vi "Split_Queue(Subvi).vi"(11 "입력 문자열":string) -> (1 "Split_Queue2_Result":string[](array[string]), 2 "Split_Queue2":string, 3 "Split_Queue3":string, 4 "Split_Queue3_Result":string[](array[string]), 5 "Split_Queue4":string, 6 "Split_Queue4_Result":string[](array[string]))   [LabVIEW 2023]
doc: "'''\n해당 함수는 입력 문자열을 분리하여 Queue2,Queue3,Queue4 값으로 분리하여 해당 Loop에 값을 전달한다. \n'''\nInput: '문자열'\n\nReturn:\n __Queue2: BDDATA(DSPEN, TRXPSEN, TRXCEN, MINTIN, BDTEMP, ENVTEMP, PRESSURE, Number\n __Queue3: SIGDATA\n __Queue4: GPSDATA(1PPS,Latitude,Longitude,Numbero"
panel:
  out "일치 + 문자열의 나머지":string
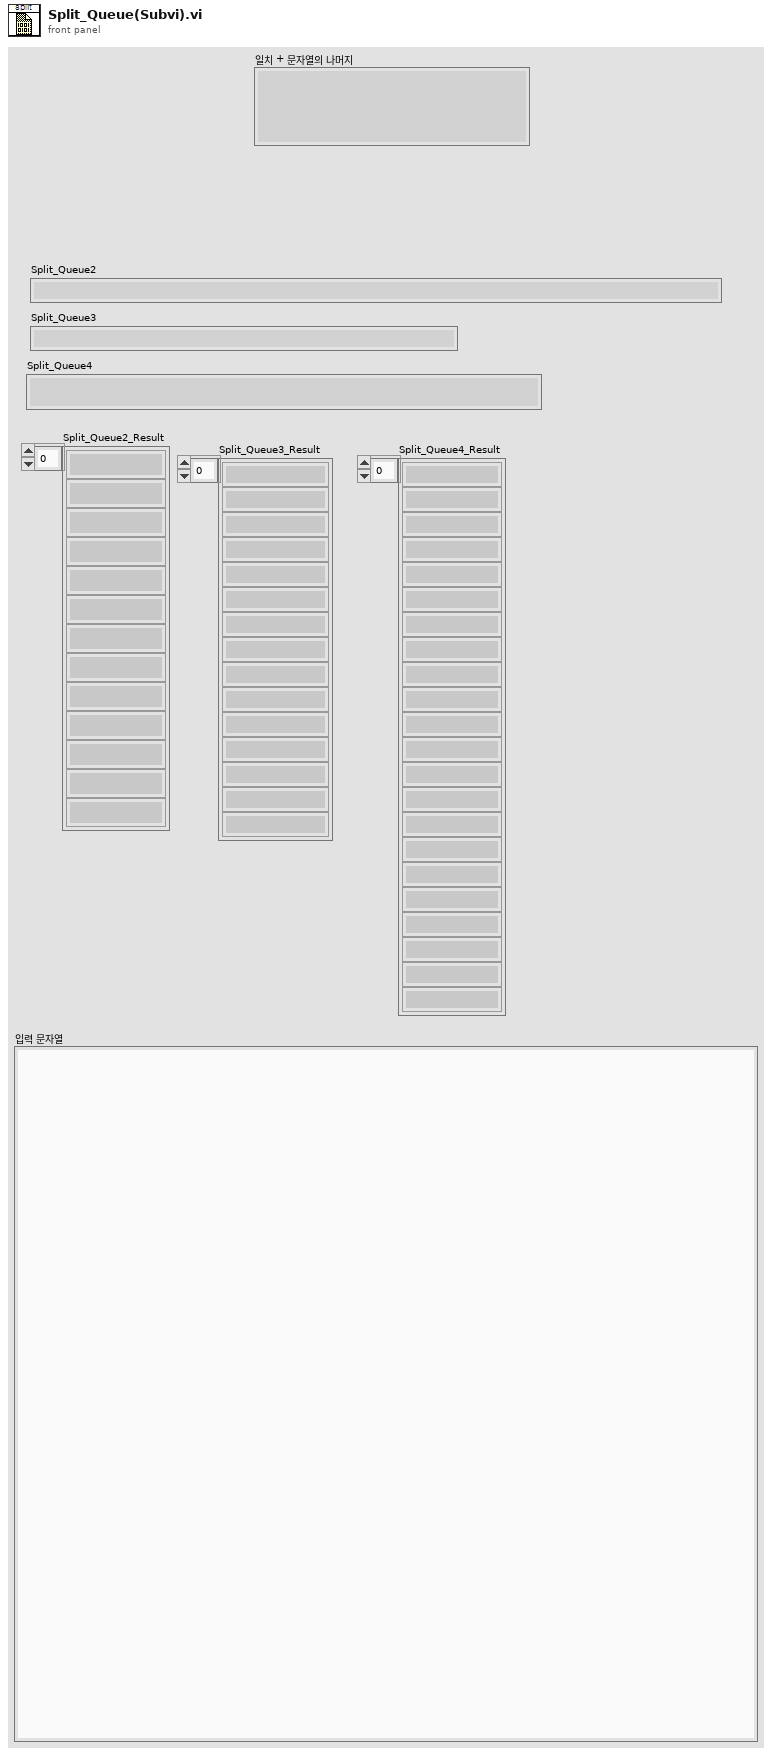
[diagram p1: front panel]
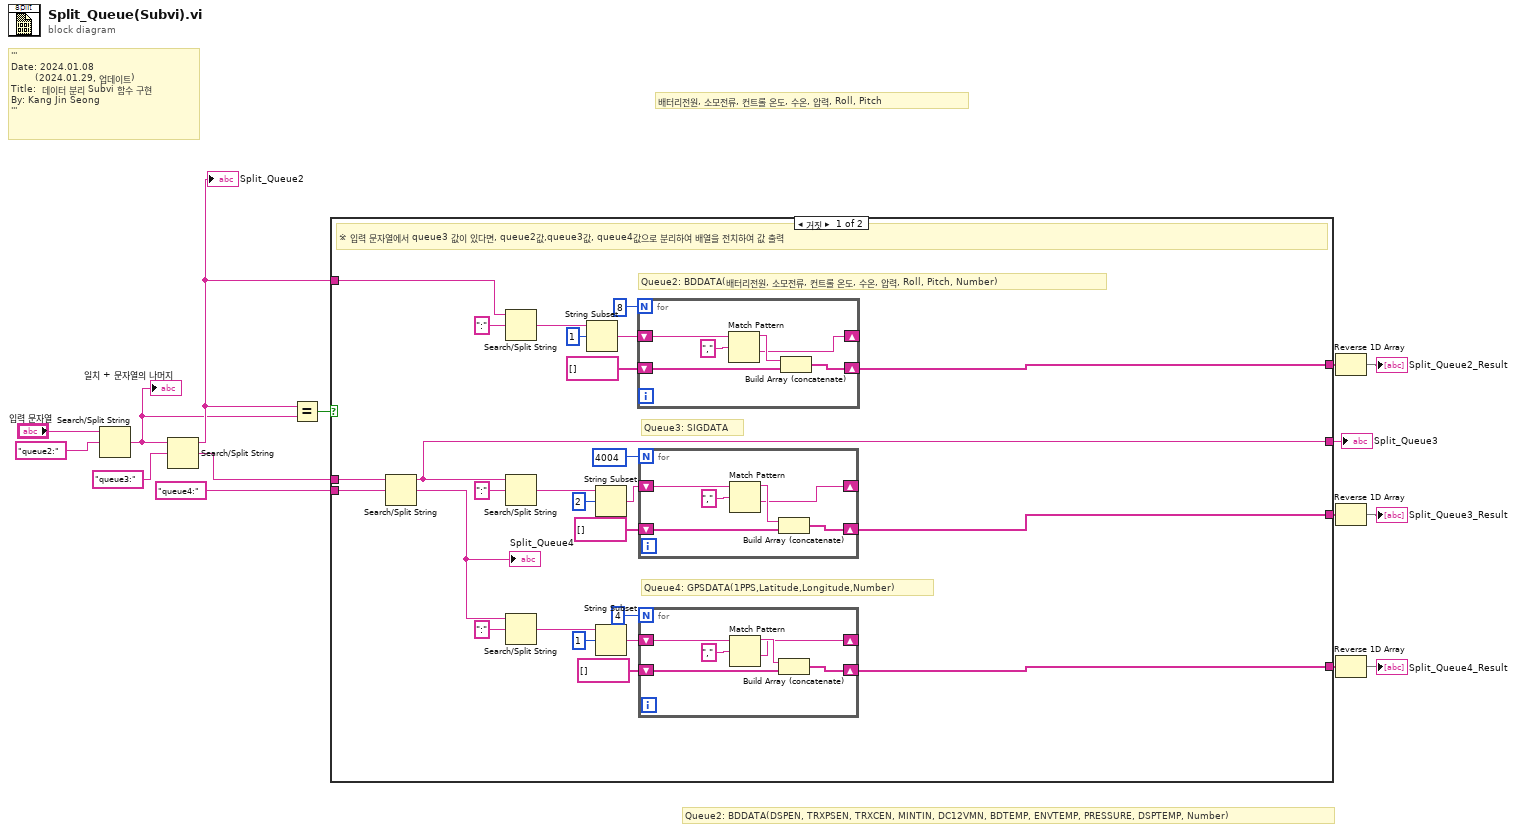
[diagram p0: block diagram]
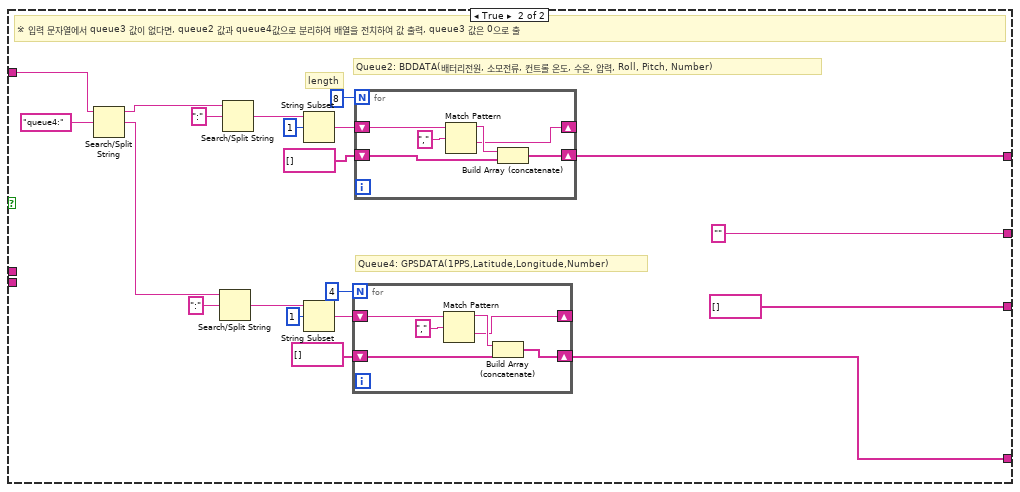
[diagram p2: hidden frame]
diagram:
  # "Queue2: BDDATA(DSPEN, TRXPSEN, TRXCEN, MINTIN, DC12VMN, BDTEMP, ENVTEMP, PRESSURE, DSPTEMP, Number)"
  # "배터리전원, 소모전류, 컨트롤 온도, 수온, 압력, Roll, Pitch"
  # "'''\nDate: 2024.01.08\n        (2024.01.29, 업데이트)\nTitle:  데이터 분리 Subvi 함수 구현\nBy: Kang Jin Seong\n'''"
  n1 = Search/Split String(string="입력 문자열", search string/char (-)="queue2:" ("검색 문자열/문자 (-)")) -> (match + rest of string=w2:string)  [unwired: 1 in, 2 out]
  "일치 + 문자열의 나머지" <- w2
  n2 = Search/Split String(string=w2, search string/char (-)="queue3:" ("검색 문자열/문자 (-)")) -> (substring before match=w3:string, match + rest of string=w7:string)  [unwired: 1 in, 1 out]
  "Split_Queue2" <- w3
  n3 = Equal?(x=w3, y=w2) -> (x = y?=w4:bool)
  n4 = case shown="거짓" w4 {
    tunnel: [w40 w60] -> w13
    tunnel: [w29 string[] []] -> w12
    tunnel: [w28 w69] -> w9
    tunnel: w3 -> [w23 w70]
    tunnel: "queue4:" ("검색 문자열/문자 (-)") -> [w21 _]
    tunnel: w7 -> [w20 _]
    tunnel: [w16 ""] -> w1
    frame False {
      # "Queue2: BDDATA(배터리전원, 소모전류, 컨트롤 온도, 수온, 압력, Roll, Pitch, Number)"
      # "Queue4: GPSDATA(1PPS,Latitude,Longitude,Number)"
      # "Queue3: SIGDATA"
      # "※ 입력 문자열에서 queue3 값이 있다면, queue2값,queue3값, queue4값으로 분리하여 배열을 전치하여 값 출력"
      n5 = Search/Split String(string=w20, search string/char (-)=w21) -> (substring before match=w16:string, match + rest of string=w41:string)  [unwired: 1 in, 1 out]
      "Split_Queue4" <- w41
      n6 = Search/Split String(string=w23, search string/char (-)=":") -> (match + rest of string=w25:string)  [unwired: 1 in, 2 out]
      n7 = Search/Split String(string=w16, search string/char (-)=":") -> (match + rest of string=w32:string)  [unwired: 1 in, 2 out]
      n8 = Search/Split String(string=w41, search string/char (-)=":") -> (match + rest of string=w37:string)  [unwired: 1 in, 2 out]
      n9 = String Subset(string=w25, offset (0)=1 ("오프셋(0)")) -> (substring=w27:string)  [unwired: 1 in]
      n10 = String Subset(string=w32, offset (0)=2 ("오프셋(0)")) -> (substring=w30:string)  [unwired: 1 in]
      n11 = String Subset(string=w37, offset (0)=1 ("오프셋(0)")) -> (substring=w39:string)  [unwired: 1 in]
      n12 = for {
        N: 8 -> [_]
        shift-right: [w56] -> _
        shift-left: w27 -> [w59]
        shift-right: [w55] -> w28
        shift-left: string[] [] -> [w54]
        n13 = Match Pattern(string=w59, regular expression="," ("정규식")) -> (before substring=w57:string, after substring=w56:string)  [unwired: 1 in, 2 out]
        n14 = Build Array (concatenate)(w57, w54) -> (w55:string[])
      }
      n15 = for {
        N: 4004 -> [_]
        shift-right: [w50] -> _
        shift-left: w30 -> [w53]
        shift-right: [w49] -> w29
        shift-left: string[] [] -> [w48]
        n16 = Match Pattern(string=w53, regular expression="," ("정규식")) -> (before substring=w51:string, after substring=w50:string)  [unwired: 1 in, 2 out]
        n17 = Build Array (concatenate)(w51, w48) -> (w49:string[])
      }
      n18 = for {
        N: 4 -> [_]
        shift-right: [w44] -> _
        shift-left: w39 -> [w47]
        shift-right: [w43] -> w40
        shift-left: string[] [] -> [w42]
        n19 = Match Pattern(string=w47, regular expression="," ("정규식")) -> (before substring=w45:string, after substring=w44:string)  [unwired: 1 in, 2 out]
        n20 = Build Array (concatenate)(w45, w42) -> (w43:string[])
      }
    }
    frame True {
      # "length"
      # "Queue2: BDDATA(배터리전원, 소모전류, 컨트롤 온도, 수온, 압력, Roll, Pitch, Number)"
      # "Queue4: GPSDATA(1PPS,Latitude,Longitude,Number)"
      # "※ 입력 문자열에서 queue3 값이 없다면, queue2 값과 queue4값으로 분리하여 배열을 전치하여 값 출력, queue3 값은 0으로 출"
      n21 = Search/Split String(string=w70, search string/char (-)="queue4:" ("검색 문자열/문자 (-)")) -> (substring before match=w62:string, match + rest of string=w61:string)  [unwired: 1 in, 1 out]
      n22 = Search/Split String(string=w61, search string/char (-)=":") -> (match + rest of string=w66:string)  [unwired: 1 in, 2 out]
      n23 = Search/Split String(string=w62, search string/char (-)=":") -> (match + rest of string=w75:string)  [unwired: 1 in, 2 out]
      n24 = String Subset(string=w75, offset (0)=1 ("오프셋(0)")) -> (substring=w77:string)  [unwired: 1 in]
      n25 = String Subset(string=w66, offset (0)=1 ("오프셋(0)")) -> (substring=w68:string)  [unwired: 1 in]
      n26 = for {
        N: 4 -> [_]
        shift-right: [w82] -> _
        shift-left: w68 -> [w85]
        shift-right: [w81] -> w60
        shift-left: string[] [] -> [w80]
        n27 = Match Pattern(string=w85, regular expression="," ("정규식")) -> (before substring=w83:string, after substring=w82:string)  [unwired: 1 in, 2 out]
        n28 = Build Array (concatenate)(w83, w80) -> (w81:string[])
      }
      n29 = for {
        N: 8 -> [_]
        shift-right: [w88] -> _
        shift-left: w77 -> [w91]
        shift-right: [w87] -> w69
        shift-left: string[] [] -> [w86]
        n30 = Match Pattern(string=w91, regular expression="," ("정규식")) -> (before substring=w89:string, after substring=w88:string)  [unwired: 1 in, 2 out]
        n31 = Build Array (concatenate)(w89, w86) -> (w87:string[])
      }
    }
  }
  "Split_Queue3" <- w1
  n32 = Reverse 1D Array(array=w9) -> (reversed array=→"Split_Queue2_Result":string[])
  n33 = Reverse 1D Array(array=w12) -> (reversed array=→"Split_Queue3_Result":string[])
  n34 = Reverse 1D Array(array=w13) -> (reversed array=→"Split_Queue4_Result":string[])
